vi "SendCerebus32.vi"(1 "String":string, 4 "Mode":T1(ring)) -> ()   [LabVIEW 2011]
uses:
  <vilib>/DAQmx/write.llb/DAQmx Write (Digital 1D Bool 1Chan 1Samp).vi
  <vilib>/DAQmx/miscellaneous.llb/DAQmx Fill In Error Info.vi
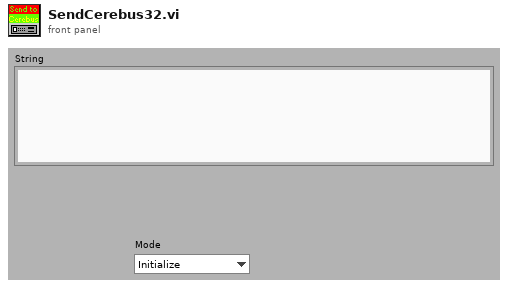
[diagram p1: front panel]
types:
  T1 = enum16{"Initialize", "String", "Start", "New Session", "Stop", "Resume", "Close"}
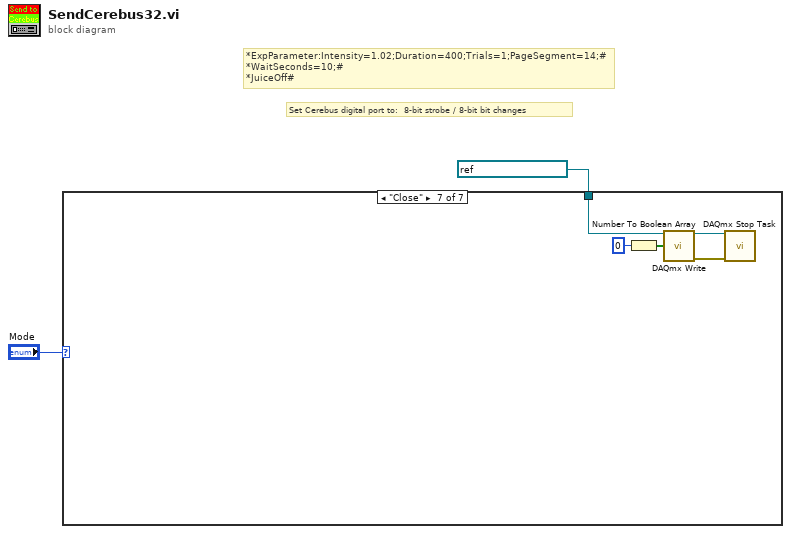
[diagram p0: block diagram]
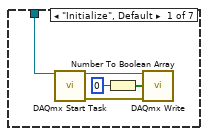
[diagram p2: hidden frame]
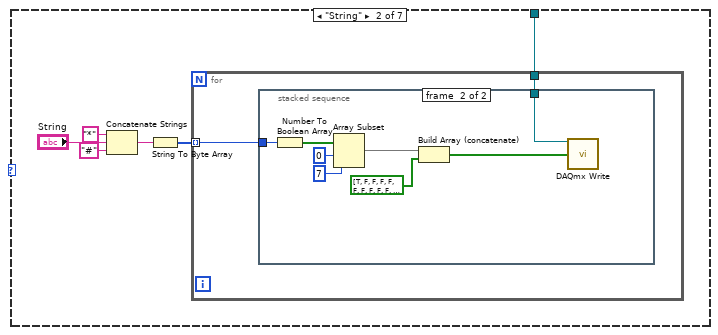
[diagram p3: hidden frame]
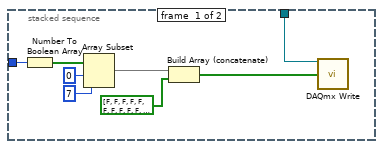
[diagram p4: hidden frame]
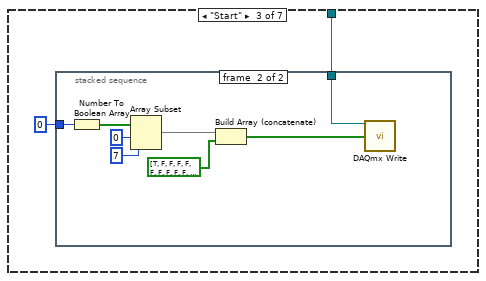
[diagram p5: hidden frame]
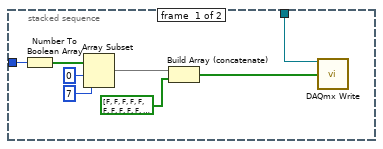
[diagram p6: hidden frame]
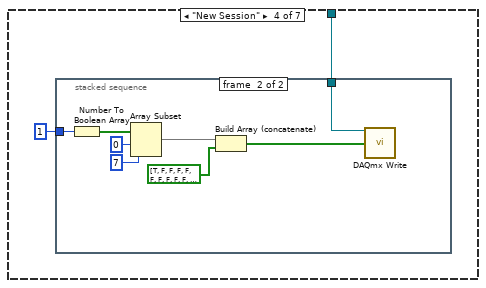
[diagram p7: hidden frame]
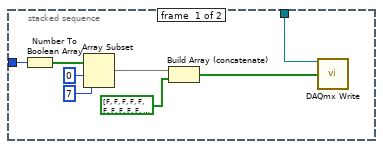
[diagram p8: hidden frame]
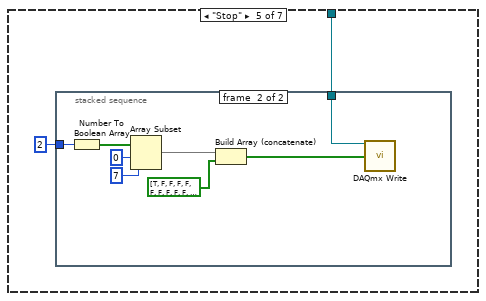
[diagram p9: hidden frame]
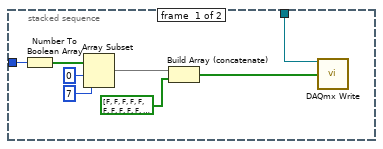
[diagram p10: hidden frame]
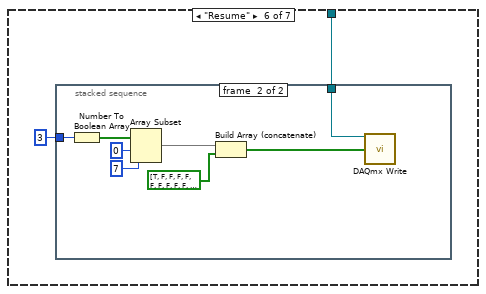
[diagram p11: hidden frame]
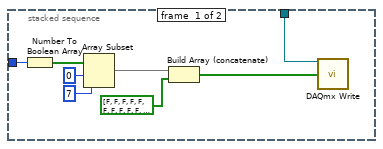
[diagram p12: hidden frame]
diagram:
  # "Set Cerebus digital port to:  8-bit strobe / 8-bit bit changes"
  # "*ExpParameter:Intensity=1.02;Duration=400;Trials=1;PageSegment=14;#\n*WaitSeconds=10;#\n*JuiceOff#"
  n1 = case shown="\"Close\"" "Mode" {
    tunnel: refnum<k21> "cerebus_markers" ("task/channels in") -> [w7 w8 w33 w51 w69 w87 w104]
    frame "Initialize", Default {
      n2 = call <vilib>:"DAQmx Start Task.vi"("task/channels in"=w7) -> ("task out"=w6:refnum<k21>, "error out"=w5:errorcluster)  [unwired: 13 in]
      n3 = Number To Boolean Array(number=u32 0) -> (Boolean array=w3:bool[])
      n4 = call-poly <vilib>:"DAQmx Write.vi"("task/channels in"=w6, "data"=w3, "error in"=w5) -> ()  [unwired: 10 in, 3 out]
    }
    frame "String" {
      n5 = Concatenate Strings("*", "String", "#" ("string")) -> (w10:string)
      n6 = String To Byte Array(string=w10) -> (unsigned byte array=w13:u8[])
      n7 = for {
        tunnel: w13 -> [w14] mode=indexing
        tunnel: w8 -> [w15]
        n8 = stacked-sequence {
          tunnel: w14 -> [w23 w25]
          tunnel: w15 -> [w22 w31]
          frame #0 {
            n9 = Number To Boolean Array(number=w23) -> (Boolean array=w21:bool[])
            n10 = Array Subset(array=w21, index=0, length=7) -> (w18:bool[])
            n11 = Build Array (concatenate)(w18, bool[] [FALSE, FALSE, FALSE, FALSE, FALSE, FALSE, FALSE, FALSE, FALSE, FALSE, FALSE, FALSE, FALSE, FALSE, FALSE, FALSE, FALSE, FALSE, FALSE, FALSE, FALSE, FALSE, FALSE, FALSE, FALSE] ("array")) -> (w16:bool[])
            n12 = call-poly <vilib>:"DAQmx Write.vi"("task/channels in"=w22, "data"=w16) -> ()  [unwired: 11 in, 3 out]
          }
          frame #1 {
            n13 = Number To Boolean Array(number=w25) -> (Boolean array=w30:bool[])
            n14 = Array Subset(array=w30, index=0, length=7) -> (w27:bool[])
            n15 = Build Array (concatenate)(w27, bool[] [TRUE, FALSE, FALSE, FALSE, FALSE, FALSE, FALSE, FALSE, FALSE, FALSE, FALSE, FALSE, FALSE, FALSE, FALSE, FALSE, FALSE, FALSE, FALSE, FALSE, FALSE, FALSE, FALSE, FALSE, FALSE] ("array")) -> (w24:bool[])
            n16 = call-poly <vilib>:"DAQmx Write.vi"("task/channels in"=w31, "data"=w24) -> ()  [unwired: 11 in, 3 out]
          }
        }
      }
    }
    frame "Start" {
      n17 = stacked-sequence {
        tunnel: u8 0 -> [w41 w43]
        tunnel: w33 -> [w40 w49]
        frame #0 {
          n18 = Number To Boolean Array(number=w41) -> (Boolean array=w39:bool[])
          n19 = Array Subset(array=w39, index=0, length=7) -> (w36:bool[])
          n20 = Build Array (concatenate)(w36, bool[] [FALSE, FALSE, FALSE, FALSE, FALSE, FALSE, FALSE, FALSE, FALSE, FALSE, FALSE, FALSE, FALSE, FALSE, FALSE, FALSE, FALSE, FALSE, FALSE, FALSE, FALSE, FALSE, FALSE, FALSE, FALSE] ("array")) -> (w34:bool[])
          n21 = call-poly <vilib>:"DAQmx Write.vi"("task/channels in"=w40, "data"=w34) -> ()  [unwired: 11 in, 3 out]
        }
        frame #1 {
          n22 = Number To Boolean Array(number=w43) -> (Boolean array=w48:bool[])
          n23 = Array Subset(array=w48, index=0, length=7) -> (w45:bool[])
          n24 = Build Array (concatenate)(w45, bool[] [TRUE, FALSE, FALSE, FALSE, FALSE, FALSE, FALSE, FALSE, FALSE, FALSE, FALSE, FALSE, FALSE, FALSE, FALSE, FALSE, FALSE, FALSE, FALSE, FALSE, FALSE, FALSE, FALSE, FALSE, FALSE] ("array")) -> (w42:bool[])
          n25 = call-poly <vilib>:"DAQmx Write.vi"("task/channels in"=w49, "data"=w42) -> ()  [unwired: 11 in, 3 out]
        }
      }
    }
    frame "New Session" {
      n26 = stacked-sequence {
        tunnel: u8 1 -> [w59 w61]
        tunnel: w51 -> [w58 w67]
        frame #0 {
          n27 = Number To Boolean Array(number=w59) -> (Boolean array=w57:bool[])
          n28 = Array Subset(array=w57, index=0, length=7) -> (w54:bool[])
          n29 = Build Array (concatenate)(w54, bool[] [FALSE, FALSE, FALSE, FALSE, FALSE, FALSE, FALSE, FALSE, FALSE, FALSE, FALSE, FALSE, FALSE, FALSE, FALSE, FALSE, FALSE, FALSE, FALSE, FALSE, FALSE, FALSE, FALSE, FALSE, FALSE] ("array")) -> (w52:bool[])
          n30 = call-poly <vilib>:"DAQmx Write.vi"("task/channels in"=w58, "data"=w52) -> ()  [unwired: 11 in, 3 out]
        }
        frame #1 {
          n31 = Number To Boolean Array(number=w61) -> (Boolean array=w66:bool[])
          n32 = Array Subset(array=w66, index=0, length=7) -> (w63:bool[])
          n33 = Build Array (concatenate)(w63, bool[] [TRUE, FALSE, FALSE, FALSE, FALSE, FALSE, FALSE, FALSE, FALSE, FALSE, FALSE, FALSE, FALSE, FALSE, FALSE, FALSE, FALSE, FALSE, FALSE, FALSE, FALSE, FALSE, FALSE, FALSE, FALSE] ("array")) -> (w60:bool[])
          n34 = call-poly <vilib>:"DAQmx Write.vi"("task/channels in"=w67, "data"=w60) -> ()  [unwired: 11 in, 3 out]
        }
      }
    }
    frame "Stop" {
      n35 = stacked-sequence {
        tunnel: u8 2 -> [w77 w79]
        tunnel: w69 -> [w76 w85]
        frame #0 {
          n36 = Number To Boolean Array(number=w77) -> (Boolean array=w75:bool[])
          n37 = Array Subset(array=w75, index=0, length=7) -> (w72:bool[])
          n38 = Build Array (concatenate)(w72, bool[] [FALSE, FALSE, FALSE, FALSE, FALSE, FALSE, FALSE, FALSE, FALSE, FALSE, FALSE, FALSE, FALSE, FALSE, FALSE, FALSE, FALSE, FALSE, FALSE, FALSE, FALSE, FALSE, FALSE, FALSE, FALSE] ("array")) -> (w70:bool[])
          n39 = call-poly <vilib>:"DAQmx Write.vi"("task/channels in"=w76, "data"=w70) -> ()  [unwired: 11 in, 3 out]
        }
        frame #1 {
          n40 = Number To Boolean Array(number=w79) -> (Boolean array=w84:bool[])
          n41 = Array Subset(array=w84, index=0, length=7) -> (w81:bool[])
          n42 = Build Array (concatenate)(w81, bool[] [TRUE, FALSE, FALSE, FALSE, FALSE, FALSE, FALSE, FALSE, FALSE, FALSE, FALSE, FALSE, FALSE, FALSE, FALSE, FALSE, FALSE, FALSE, FALSE, FALSE, FALSE, FALSE, FALSE, FALSE, FALSE] ("array")) -> (w78:bool[])
          n43 = call-poly <vilib>:"DAQmx Write.vi"("task/channels in"=w85, "data"=w78) -> ()  [unwired: 11 in, 3 out]
        }
      }
    }
    frame "Resume" {
      n44 = stacked-sequence {
        tunnel: u8 3 -> [w95 w97]
        tunnel: w87 -> [w94 w103]
        frame #0 {
          n45 = Number To Boolean Array(number=w95) -> (Boolean array=w93:bool[])
          n46 = Array Subset(array=w93, index=0, length=7) -> (w90:bool[])
          n47 = Build Array (concatenate)(w90, bool[] [FALSE, FALSE, FALSE, FALSE, FALSE, FALSE, FALSE, FALSE, FALSE, FALSE, FALSE, FALSE, FALSE, FALSE, FALSE, FALSE, FALSE, FALSE, FALSE, FALSE, FALSE, FALSE, FALSE, FALSE, FALSE] ("array")) -> (w88:bool[])
          n48 = call-poly <vilib>:"DAQmx Write.vi"("task/channels in"=w94, "data"=w88) -> ()  [unwired: 11 in, 3 out]
        }
        frame #1 {
          n49 = Number To Boolean Array(number=w97) -> (Boolean array=w102:bool[])
          n50 = Array Subset(array=w102, index=0, length=7) -> (w99:bool[])
          n51 = Build Array (concatenate)(w99, bool[] [TRUE, FALSE, FALSE, FALSE, FALSE, FALSE, FALSE, FALSE, FALSE, FALSE, FALSE, FALSE, FALSE, FALSE, FALSE, FALSE, FALSE, FALSE, FALSE, FALSE, FALSE, FALSE, FALSE, FALSE, FALSE] ("array")) -> (w96:bool[])
          n52 = call-poly <vilib>:"DAQmx Write.vi"("task/channels in"=w103, "data"=w96) -> ()  [unwired: 11 in, 3 out]
        }
      }
    }
    frame "Close" {
      n53 = Number To Boolean Array(number=u32 0) -> (Boolean array=w107:bool[])
      n54 = call-poly <vilib>:"DAQmx Write.vi"("task/channels in"=w104, "data"=w107) -> ("task out"=w106:refnum<k21>, "error out"=w105:errorcluster)  [unwired: 11 in, 1 out]
      n55 = call <vilib>:"DAQmx Stop Task.vi"("task/channels in"=w106, "error in"=w105) -> ()  [unwired: 12 in, 2 out]
    }
  }
